vi "main.vi"() -> ()   [LabVIEW 2023]
uses:
  state-machine-states.ctl
  tab-control-states.ctl
  <vilib>/DAQmx/read.llb/DAQmx Read (Analog DBL 1Chan 1Samp).vi
  <vilib>/DAQmx/create/channels.llb/DAQmx Create Channel (AI-Temperature-Thermocouple).vi
  <vilib>/DAQmx/miscellaneous.llb/DAQmx Fill In Error Info.vi
  bronkhorst_flow-bus/Bronkhorst FLOW-BUS/Public/Data/Measure/Read Measure (Direct).vi
  bronkhorst_flow-bus/Bronkhorst FLOW-BUS/Public/Configure/Setpoint/Configure Setpoint (Percentage).vi
  bronkhorst_flow-bus/Bronkhorst FLOW-BUS/Public/Data/Setpoint/Read Setpoint (Percentage).vi
  bronkhorst_flow-bus/Bronkhorst FLOW-BUS/Public/Data/Measure/Read Measure (Percentage).vi
  bronkhorst_flow-bus/Bronkhorst FLOW-BUS/Bronkhorst FLOW-BUS.lvlib
panel:
  in  "Stop":bool
  in  "pause":bool
  in  "exit":bool
  out "state":T1
  out "error out":errorcluster
  out "Status":string
  in  "Tab Control":enum32{"setup", "run", "graphs", "errors"}(tab)
  in  "Start":bool
  in  "MFC 1":refnum<visa-resource-name>="COM31"
  in  "MFC 2":refnum<visa-resource-name>="COM32"
  in  "MFM 3":refnum<visa-resource-name>="COM33"
  in  "MFM 4":refnum<visa-resource-name>="COM34"
  in  "TC1 Channel":tag="cDAQ1Mod1/ai0"
  out "MFM4 (ml/min) 2":dbl caption="Measure Percentage"
  out "Measure (ml/min)":dbl caption="Measure Percentage"
  out "Measure (%) 2":dbl caption="Measure Percentage"
  in  "Setpoint  (%) 2":dbl min=0.0 max=100.0 step=1.0 format="%#.2g"
  out "Setpoint Percentage 2":dbl caption="Setpoint Percentage" format="%#g"
  out "Measure (%)":dbl caption="Measure Percentage"
  in  "Setpoint  (%)":dbl min=0.0 max=100.0 step=1.0 format="%#.2g"
  out "Setpoint Percentage":dbl format="%#g"
  out "TC1 (degC)":dbl format="%0.2f"
  out "MFM Sensor History":dbl[][](graph)
  out "Temperature Sensor History":dbl[](graph)
  out "errors":errorcluster
  in  "Clear Errors":bool
  # "Usage Instructions:\n\n1. Select \"setup\" tab, ensure correct \n    COM port & Channel for each device\n\n2. To start Data Aquisition press \"Start\" button\n\n3. Select Setpoint for MFC1 & MFC2\n\n4. View Graphs in \"graphs\" tab\n\n5. Pause and Unpause data aquisition with \"pause\" button\n\n6. To export data to Excel, right click on topmost graph view \n     and select:\n     - \"Export\" -> \"Export  Data to Excel\"\n     - Name & Save Excel file\n        (Note: All data will be exported not just \"active\" plots)\n\n\n7. To Clear sensor history press \"Stop\" button\n     - While stopped, setup controls are available\n\n8. To Exit program, click \"Exit\" Button\n\n9. If Error shows, attempt to remedy error then press\n     \"clear error\" button. Program will revert to Setup"
  # "Percentage"
  # "Gas  \nOut"
  # "Nitrogen \nIn"
  # "Ammonia \nIn"
  # "Gas  \nOut"
  # "MFC2"
  # "MFM4"
  # "MFM3"
  # "MFC1"
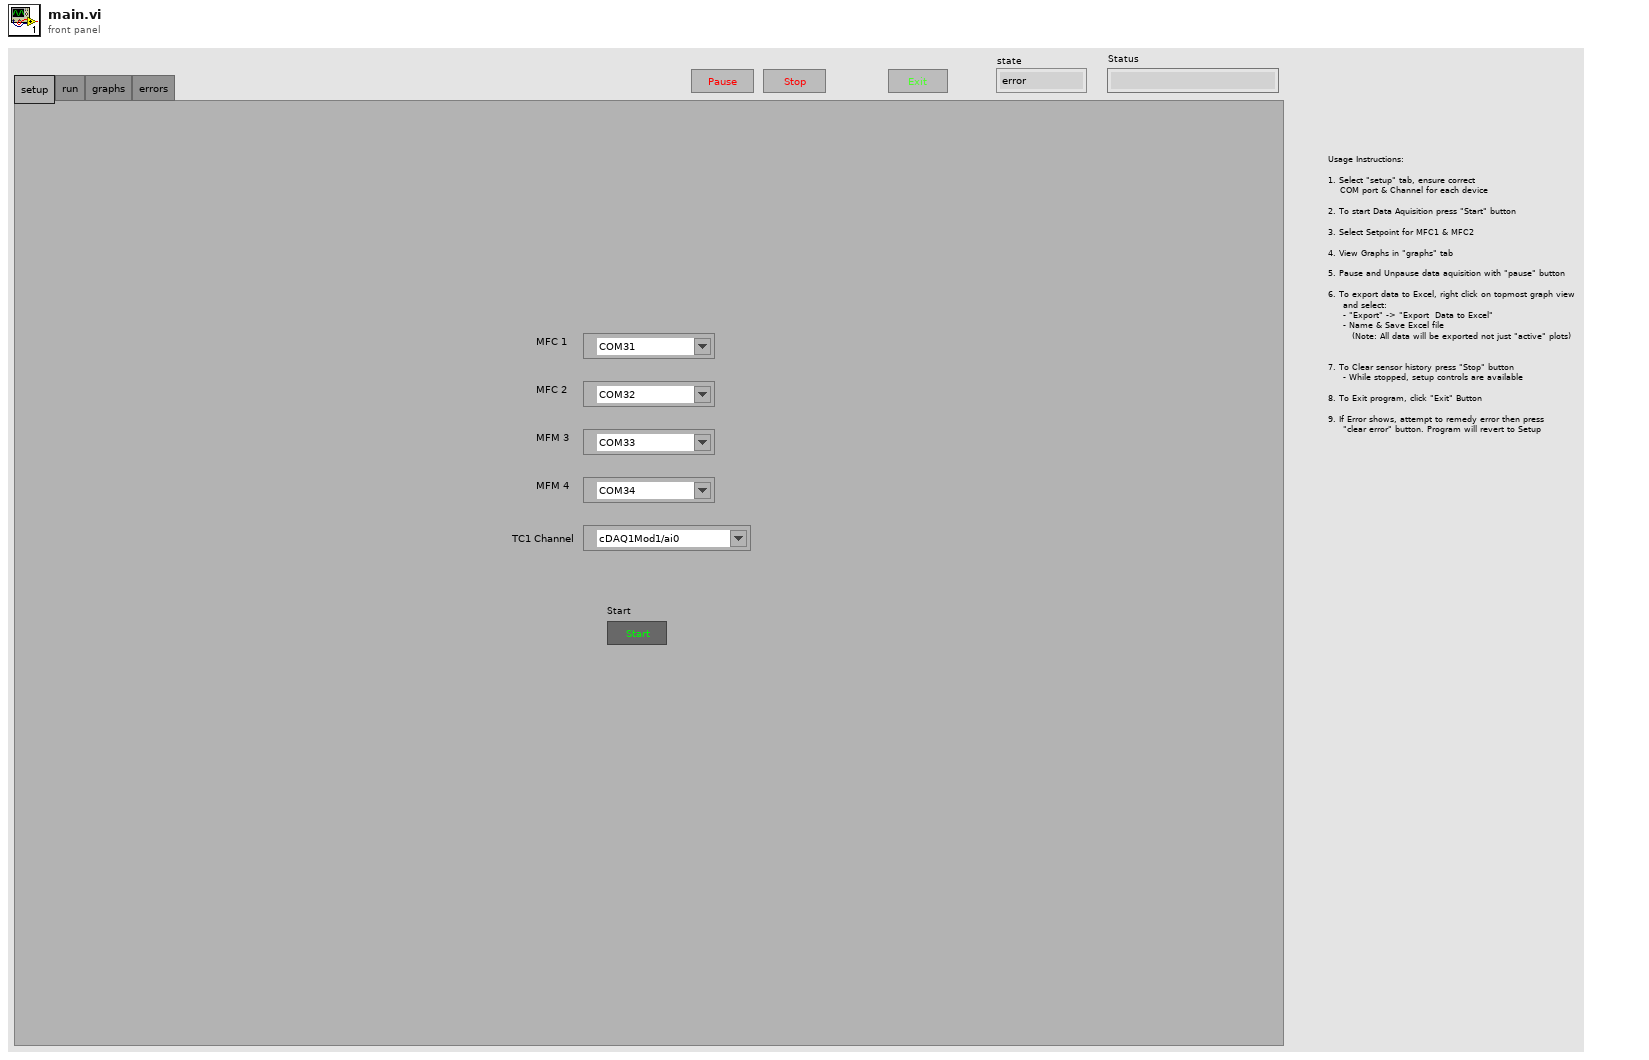
[diagram p1: front panel]
types:
  T1 = typedef "state-machine-states.ctl" = enum16{"error", "wait", "init", "start", "run", "stop", "clear-error", "shutdown"}
  T2 = enum8{"Enabled", "Disabled", "Disabled and Grayed Out"}
  T3 = typedef "tab-control-states.ctl" = enum32{"setup", "run", "graphs", "errors"}
  T4 = enum32{"BUS/RS232", "Analog input", "FLOW-BUS slave", "Valve close", "Controller idle", "Testing mode", "Tuning mode", "Setpoint 100%", "Valve fully open", "Calibration mode", "Analog slave", "Keyboard or FLOW-BUS setpoint", "Setpoint 0%", "FLOW-BUS analog slave", "(FPP) Range select mode", "(FPP) Manual start sensor select, automatic end sensor", "(FPP) Automatic start sensor select, manual end sensor", "(FPP) Automatic start and end sensor", "RS232 Setpoint", "RS232 broadcast mode", "Valve stearing (valve = setpoint)", "Analog valve stearing (valve = analog setpoint)", "Valve safe state"}
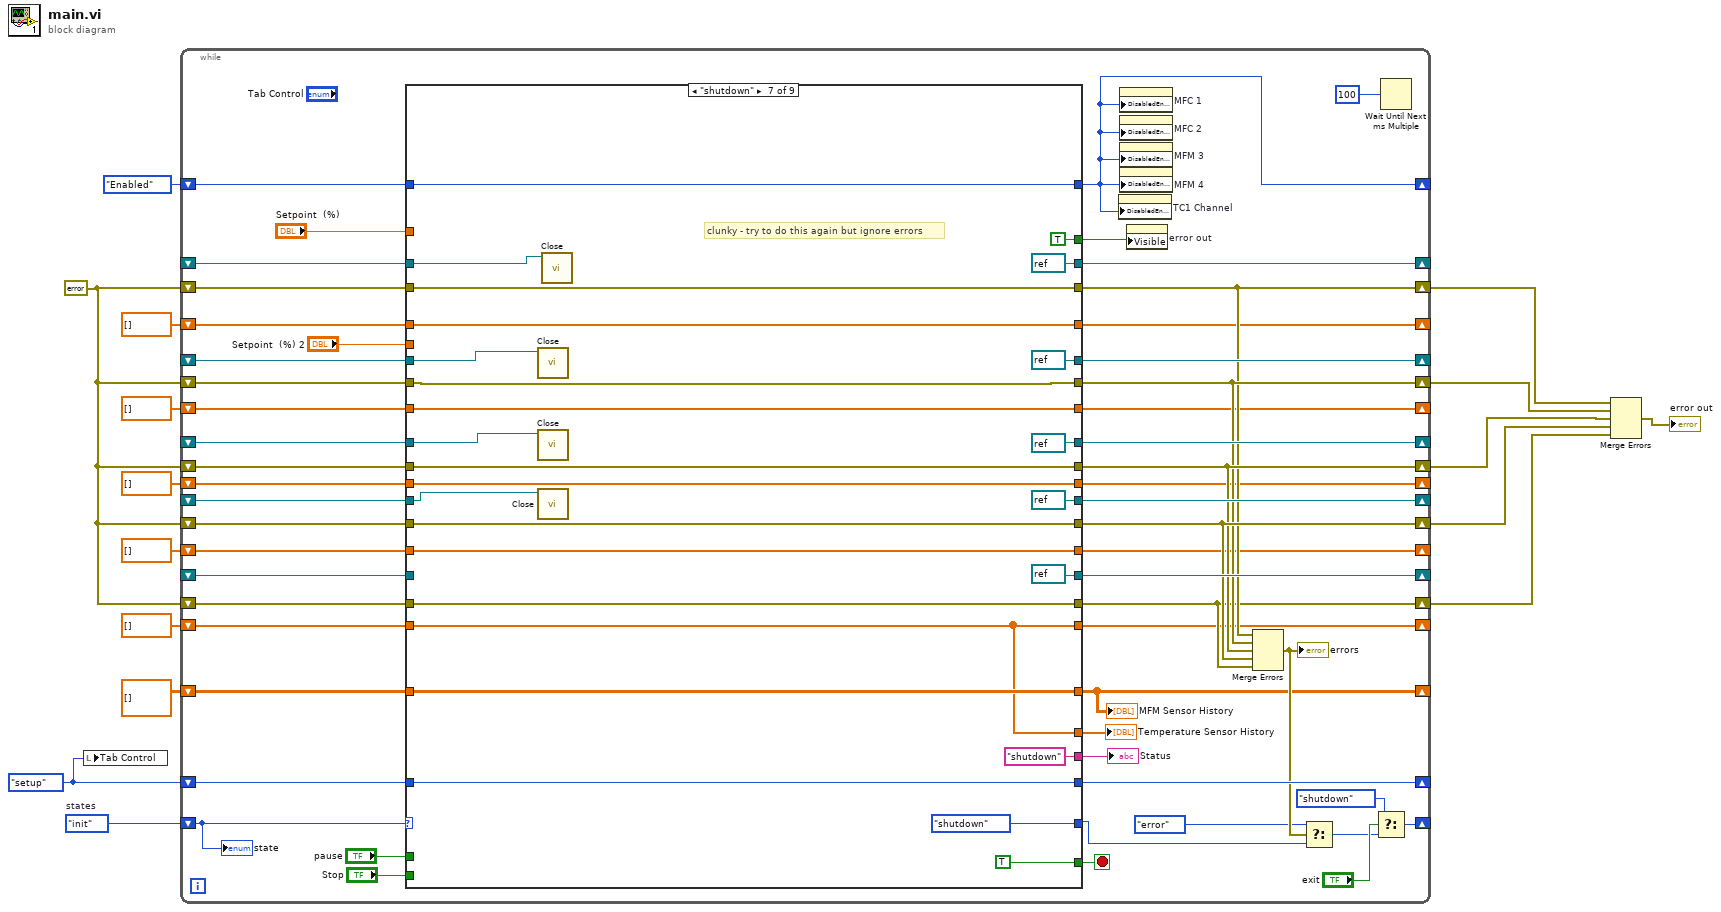
[diagram p0: block diagram]
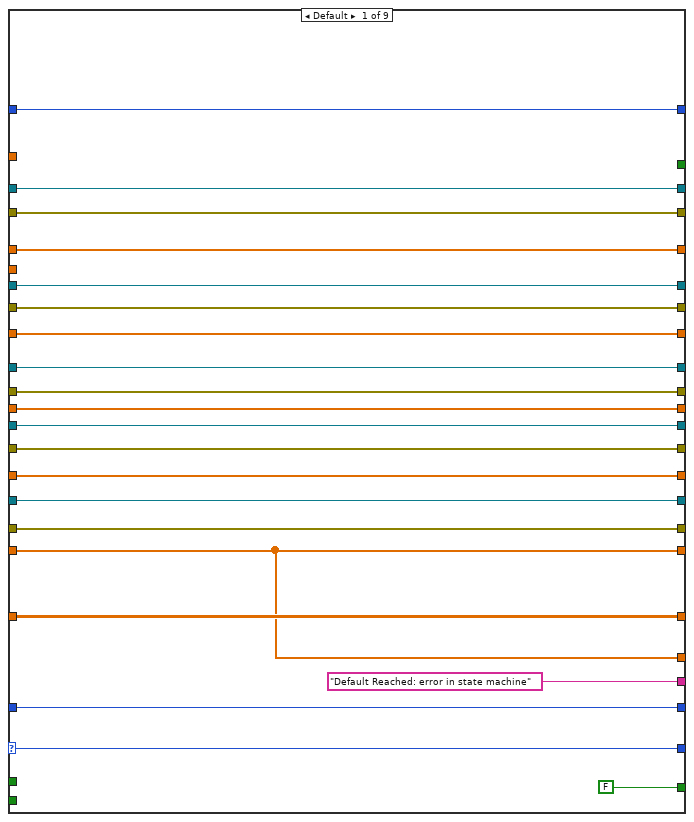
[diagram p2: hidden frame]
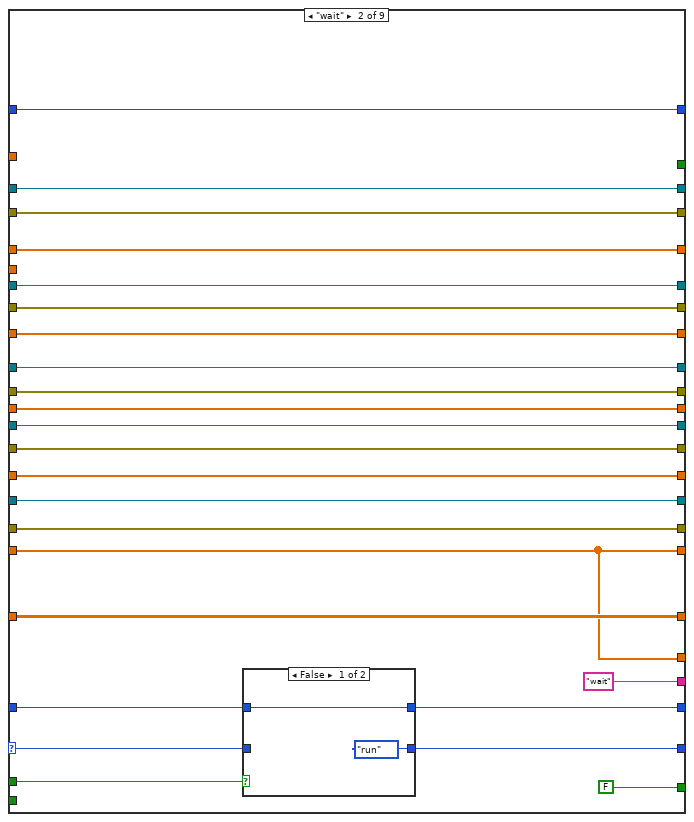
[diagram p3: hidden frame]
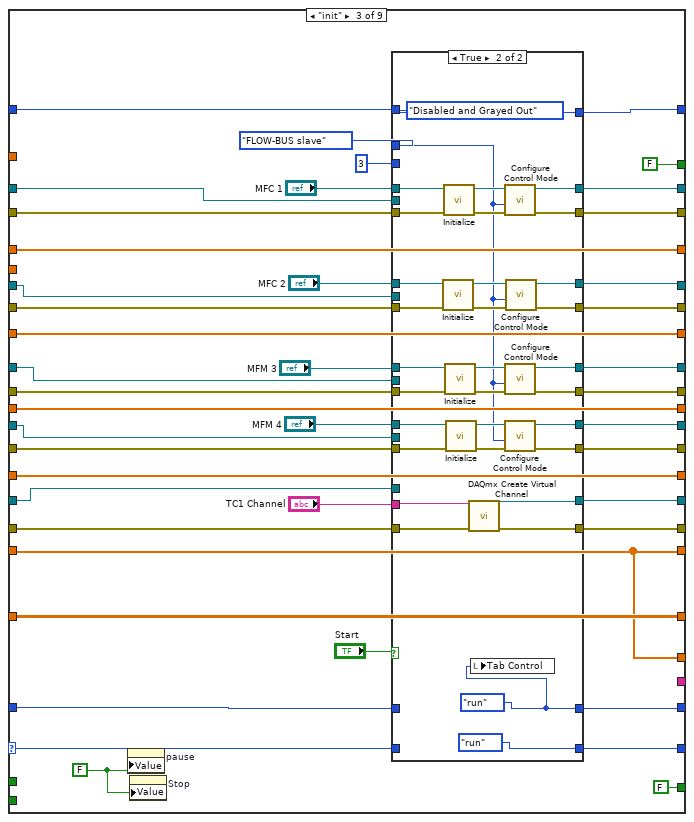
[diagram p5: hidden frame]
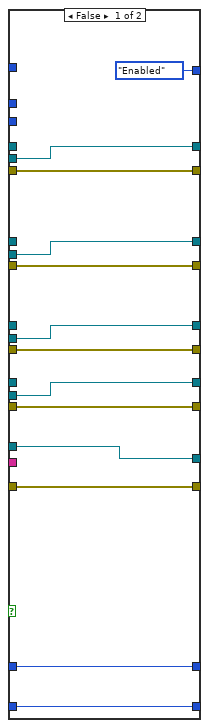
[diagram p6: hidden frame]
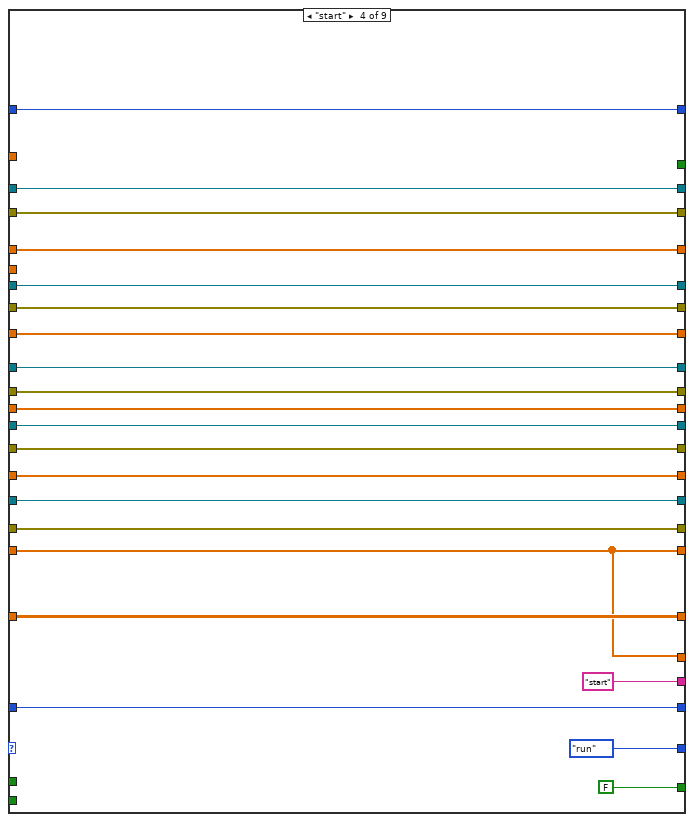
[diagram p7: hidden frame]
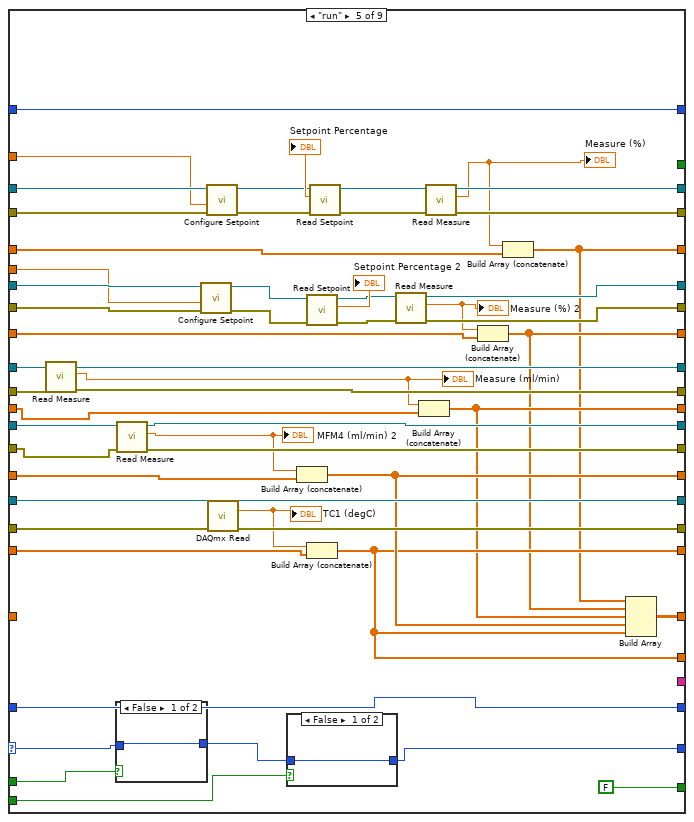
[diagram p8: hidden frame]
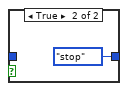
[diagram p9: hidden frame]
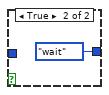
[diagram p10: hidden frame]
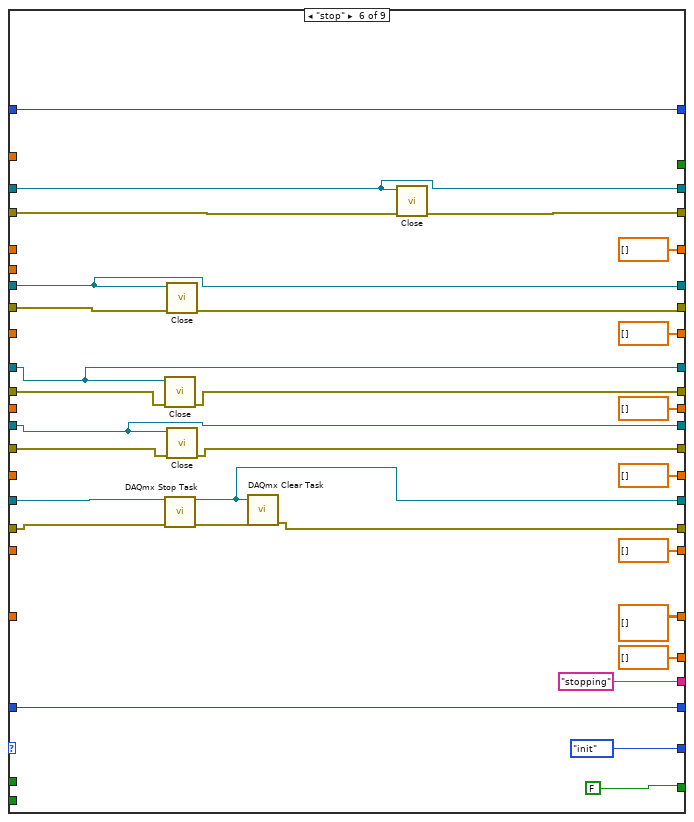
[diagram p11: hidden frame]
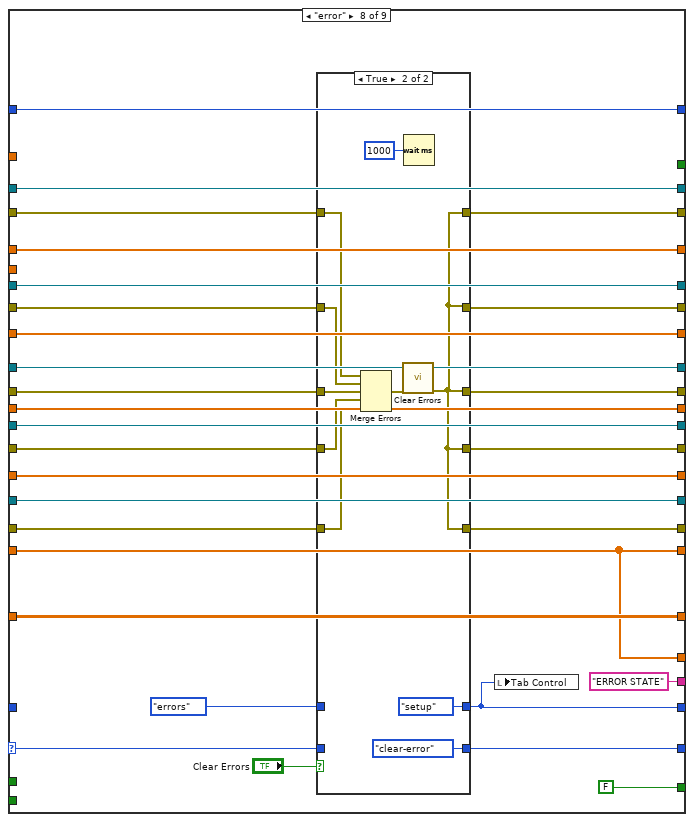
[diagram p12: hidden frame]
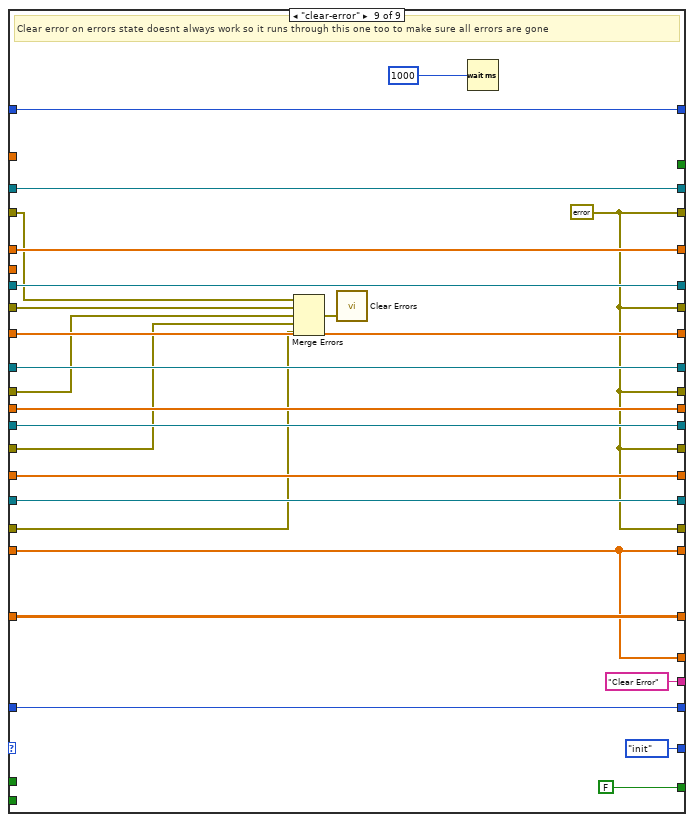
[diagram p14: hidden frame]
diagram:
  w9 = errorcluster {"status"=FALSE, "code"=0, "source"=""} ("error out")
  w10 = state-machine-states."init"  # states
  w7 = tab-control-states."setup" ("Tab Control")
  n1 = local write "Tab Control"(w7) -> ()
  n2 = while {
    shift-right: [w52] -> _
    shift-left: w7 -> [w39]
    shift-right: [w69] -> _
    shift-left: _ -> [w61]
    shift-right: [w44] -> w15
    shift-left: w9 -> [w65]
    shift-right: [w68] -> _
    shift-left: _ -> [w60]
    shift-right: [w45] -> w14
    shift-left: w9 -> [w64]
    shift-right: [w67] -> _
    shift-left: _ -> [w59]
    shift-right: [w46] -> w13
    shift-left: w9 -> [w63]
    shift-right: [w66] -> _
    shift-left: _ -> [w58]
    shift-right: [w47] -> w12
    shift-left: w9 -> [w62]
    shift-right: [w57] -> _
    shift-left: _ -> [w56]
    shift-right: [w43] -> w11
    shift-left: w9 -> [w55]
    shift-right: [w36] -> _
    shift-left: w10 -> [w50]
    shift-right: [w40] -> _
    shift-left: T2."Enabled" ("Disabled") -> [w41]
    shift-right: [w30] -> _
    shift-left: sgl[] [] -> [w29]
    shift-right: [w28] -> _
    shift-left: dbl[] [] -> [w27]
    shift-right: [w25] -> _
    shift-left: sgl[] [] -> [w24]
    shift-right: [w23] -> _
    shift-left: dbl[] [] -> [w22]
    shift-right: [w21] -> _
    shift-left: dbl[] [] -> [w20]
    shift-right: [w19] -> _
    shift-left: dbl[][] [] -> [w18]
    stop <- w34 stop-if-true
    n3 = case shown="\"shutdown\"" w50 {
      selector: w50 -> [w78 w98 w159 _ w251 _ _ w355 _]
      tunnel: [w80 w99 w127 w217 w248 w313 w341 w353 w389] -> w52
      tunnel: w39 -> [w80 w100 w160 w217 w248 w313 w341 _ w389]
      tunnel: [w90 w114 w139 w227 w272 w298 refnum<visa-resource-name> refnum ("VISA resource name out") w371 w412] -> w69
      tunnel: [w89 w113 w140 w226 w271 w315 w334 w347 w391] -> w44
      tunnel: [w87 w104 w145 w225 w266 w300 refnum<visa-resource-name> refnum ("VISA resource name out") w370 w411] -> w68
      tunnel: [w88 w105 w146 w224 w267 w301 w328 w346 w391] -> w45
      tunnel: [w86 w106 w151 w223 w258 w306 refnum<visa-resource-name> refnum ("VISA resource name out") w369 w410] -> w67
      tunnel: [w85 w107 w152 w222 w259 w307 w327 w345 w391] -> w46
      tunnel: [w84 w108 w155 w221 w255 w303 refnum<visa-resource-name> refnum ("VISA resource name out") w368 w409] -> w66
      tunnel: [w83 w109 w156 w220 w254 w302 w326 w344 w391] -> w47
      tunnel: w65 -> [w89 w113 w142 w226 w270 w299 w334 w352 w396]
      tunnel: w64 -> [w88 w105 w148 w224 w268 w305 w328 w351 w395]
      tunnel: w63 -> [w85 w107 w150 w222 w260 w308 w327 w350 w394]
      tunnel: w62 -> [w83 w109 w154 w220 w256 w304 w326 w349 w393]
      tunnel: w61 -> [w90 w114 w131 w227 w273 w298 w338 w371 w412]
      tunnel: w60 -> [w87 w104 w132 w225 w269 w300 w337 w370 w411]
      tunnel: w59 -> [w86 w106 w130 w223 w261 w306 w336 w369 w410]
      tunnel: w58 -> [w84 w108 w133 w221 w257 w303 w335 w368 w409]
      tunnel: [w82 w110 w135 w219 w263 w309 refnum<k21> refnum ("task out") w367 w408] -> w57
      tunnel: w56 -> [w82 w110 w138 w219 w265 w312 _ w367 w408]
      tunnel: [w81 w111 w134 w218 w262 w310 w325 w343 w391] -> w43
      tunnel: w55 -> [w81 w111 w136 w218 w264 w311 w325 w348 w392]
      tunnel: "Setpoint  (%)" -> [_ _ _ _ w253 _ _ _ _]
      tunnel: "Setpoint  (%) 2" -> [_ _ _ _ w252 _ _ _ _]
      tunnel: ["Default Reached: error in state machine" ("Status") "wait" ("Status") _ "start" ("Status") _ "stopping" ("Status") "shutdown" ("Status") "ERROR STATE" ("Status") "Clear Error" ("Status")] -> w51
      tunnel: [w78 w97 w158 state-machine-states."run" ("Enum") w244 state-machine-states."init" ("Enum") state-machine-states."shutdown" ("Enum") w356 state-machine-states."init"] -> w32
      tunnel: [FALSE ("x") FALSE ("x") FALSE ("x") FALSE ("x") FALSE ("x") FALSE ("x") TRUE ("x") FALSE ("x") FALSE ("x")] -> w34
      tunnel: [w76 w102 w129 w213 w249 w295 w339 w365 w406] -> w40
      tunnel: w41 -> [w76 w102 w128 w213 w249 w295 w339 w365 w406]
      tunnel: "pause" -> [_ w101 _ _ w247 _ _ _ _]
      tunnel: "Stop" -> [_ _ _ _ w246 _ _ _ _]
      tunnel: [w71 w92 w121 w212 w241 dbl[][] [] w323 w360 w401] -> w19
      tunnel: [w75 w94 w125 w211 w238 sgl[] [] w321 w361 w402] -> w30
      tunnel: w29 -> [w75 w94 w125 w211 w240 _ w321 w361 w402]
      tunnel: [w70 w91 w120 w207 w237 dbl[] [] w322 w359 w400] -> w28
      tunnel: w27 -> [w70 w91 w120 w207 w239 _ w322 w359 w400]
      tunnel: [w70 w91 w120 w207 w237 dbl[] [] w322 w359 w400] -> w26
      tunnel: [w74 w93 w124 w210 w230 sgl[] [] w320 w362 w403] -> w25
      tunnel: w24 -> [w74 w93 w124 w210 w235 _ w320 w362 w403]
      tunnel: [w73 w95 w123 w209 w229 dbl[] [] w319 w363 w404] -> w23
      tunnel: w22 -> [w73 w95 w123 w209 w233 _ w319 w363 w404]
      tunnel: [w72 w96 w122 w208 w228 dbl[] [] w318 w364 w405] -> w21
      tunnel: w20 -> [w72 w96 w122 w208 w232 _ w318 w364 w405]
      tunnel: w18 -> [w71 w92 w121 w212 _ _ w323 w360 w401]
      tunnel: [_ _ FALSE ("Visible") _ _ _ TRUE ("Visible") _ _] -> w17
      frame Default {
      }
      frame "wait" {
        n4 = case shown="False" w101 {
          tunnel: w98 -> [_ w117]
          tunnel: w100 -> [w116 w118]
          tunnel: [w116 w118] -> w99
          tunnel: [state-machine-states."run" w117] -> w97
          frame False {
          }
          frame True {
          }
        }
      }
      frame "init" {
        w126 = FALSE ("pause")
        n5 = property on="pause" class="Bool (strict)"("Value"=w126) -> ()  [unwired: 2 in, 2 out]
        n6 = property on="Stop" class="Bool (strict)"("Value"=w126) -> ()  [unwired: 2 in, 2 out]
        n7 = case shown="True" "Start" {
          tunnel: [w165 w175] -> w127
          tunnel: w160 -> [w165 _]
          tunnel: w159 -> [w164 _]
          tunnel: [w164 state-machine-states."run" ("Enum")] -> w158
          tunnel: [w169 w206] -> w156
          tunnel: [w174 w205] -> w155
          tunnel: w154 -> [w169 w204]
          tunnel: "MFM 4" -> [_ w203]
          tunnel: [w168 w200] -> w152
          tunnel: [w171 w199] -> w151
          tunnel: w150 -> [w168 w198]
          tunnel: "MFM 3" -> [_ w197]
          tunnel: w148 -> [w167 w192]
          tunnel: "MFC 2" -> [_ w191]
          tunnel: [w167 w190] -> w146
          tunnel: [w173 w189] -> w145
          tunnel: T4."FLOW-BUS slave" ("Control Mode (0: BUS/RS232)") -> [_ w179]
          tunnel: u8 3 ("Node (3)") -> [_ _]
          tunnel: w142 -> [w166 w186]
          tunnel: "MFC 1" -> [_ w185]
          tunnel: [w166 w184] -> w140
          tunnel: [w172 w183] -> w139
          tunnel: w138 -> [w162 _]
          tunnel: "TC1 Channel" -> [_ w177]
          tunnel: w136 -> [w170 w182]
          tunnel: [w162 w181] -> w135
          tunnel: [w170 w180] -> w134
          tunnel: w133 -> [w174 _]
          tunnel: w132 -> [w173 _]
          tunnel: w131 -> [w172 _]
          tunnel: w130 -> [w171 _]
          tunnel: [T2."Enabled" ("Disabled") T2."Disabled and Grayed Out" ("Disabled")] -> w129
          tunnel: w128 -> [_ _]
          frame False {
          }
          frame True {
            w175 = tab-control-states."run" ("Tab Control")
            n8 = call "Initialize.vi"("error in (no error)"=w192, "VISA resource name"=w191) -> ("error out"=w193:errorcluster, "VISA resource name out"=w194:refnum<visa-resource-name>)  [unwired: 8 in]
            n9 = call "Initialize.vi"("error in (no error)"=w186, "VISA resource name"=w185) -> ("error out"=w187:errorcluster, "VISA resource name out"=w188:refnum<visa-resource-name>)  [unwired: 8 in]
            n10 = call "Initialize.vi"("error in (no error)"=w198, "VISA resource name"=w197) -> ("error out"=w196:errorcluster, "VISA resource name out"=w195:refnum<visa-resource-name>)  [unwired: 8 in]
            n11 = call "Initialize.vi"("error in (no error)"=w204, "VISA resource name"=w203) -> ("error out"=w202:errorcluster, "VISA resource name out"=w201:refnum<visa-resource-name>)  [unwired: 8 in]
            n12 = call-poly <vilib>:"DAQmx Create Virtual Channel.vi"("physical channels"=w177, "error in"=w182) -> ("task out"=w181:refnum<k21>, "error out"=w180:errorcluster)  [unwired: 12 in]
            n13 = local write "Tab Control"(w175) -> ()
            n14 = call "Configure Control Mode.vi"("error in (no error)"=w187, "Control Mode (0: BUS/RS232)"=w179, "VISA resource name"=w188) -> ("error out"=w184:errorcluster, "VISA resource name out"=w183:refnum<visa-resource-name>)  [unwired: 7 in]
            n15 = call "Configure Control Mode.vi"("error in (no error)"=w196, "Control Mode (0: BUS/RS232)"=w179, "VISA resource name"=w195) -> ("error out"=w200:errorcluster, "VISA resource name out"=w199:refnum<visa-resource-name>)  [unwired: 7 in]
            n16 = call "Configure Control Mode.vi"("error in (no error)"=w202, "Control Mode (0: BUS/RS232)"=w179, "VISA resource name"=w201) -> ("error out"=w206:errorcluster, "VISA resource name out"=w205:refnum<visa-resource-name>)  [unwired: 7 in]
            n17 = call "Configure Control Mode.vi"("error in (no error)"=w193, "Control Mode (0: BUS/RS232)"=w179, "VISA resource name"=w194) -> ("error out"=w190:errorcluster, "VISA resource name out"=w189:refnum<visa-resource-name>)  [unwired: 7 in]
          }
        }
      }
      frame "start" {
      }
      frame "run" {
        n18 = call-poly "Read Measure.vi"("error in (no error)"=w260, "VISA resource name"=w261) -> ("error out"=w259:errorcluster, "Measure Direct"=w236:sgl, "VISA resource name out"=w258:refnum<visa-resource-name>)  [unwired: 7 in]
        "Measure (ml/min)" <- w236
        n19 = case shown="False" w247 {
          tunnel: w251 -> [w286 _]
          tunnel: [w286 state-machine-states."wait"] -> w245
          frame False {
          }
          frame True {
          }
        }
        n20 = call-poly "Read Measure.vi"("error in (no error)"=w256, "VISA resource name"=w257) -> ("error out"=w254:errorcluster, "Measure Direct"=w243:sgl, "VISA resource name out"=w255:refnum<visa-resource-name>)  [unwired: 7 in]
        "MFM4 (ml/min) 2" <- w243
        n21 = call-poly "Configure Setpoint.vi"("error in (no error)"=w268, "Setpoint Percentage (0%)"=w252, "VISA resource name"=w269) -> ("error out"=w280:errorcluster, "VISA resource name out"=w279:refnum<visa-resource-name>)  [unwired: 7 in]
        n22 = call-poly "Configure Setpoint.vi"("error in (no error)"=w270, "Setpoint Percentage (0%)"=w253, "VISA resource name"=w273) -> ("error out"=w276:errorcluster, "VISA resource name out"=w274:refnum<visa-resource-name>)  [unwired: 7 in]
        n23 = call-poly <vilib>:"DAQmx Read.vi"("task/channels in"=w265, "error in"=w264) -> ("task out"=w263:refnum<k21>, "data"=w242:dbl, "error out"=w262:errorcluster)  [unwired: 11 in]
        "TC1 (degC)" <- w242
        n24 = case shown="False" w246 {
          tunnel: w245 -> [w284 _]
          tunnel: [w284 state-machine-states."stop"] -> w244
          frame False {
          }
          frame True {
          }
        }
        n25 = Build Array (concatenate)(w243, w240) -> (w238:sgl[])
        n26 = call-poly "Read Setpoint.vi"("error in (no error)"=w280, "VISA resource name"=w279) -> ("error out"=w282:errorcluster, "Setpoint Percentage"=→"Setpoint Percentage 2":dbl, "VISA resource name out"=w281:refnum<visa-resource-name>)  [unwired: 7 in]
        n27 = Build Array (concatenate)(w242, w239) -> (w237:dbl[])
        n28 = call-poly "Read Setpoint.vi"("error in (no error)"=w276, "VISA resource name"=w274) -> ("error out"=w278:errorcluster, "Setpoint Percentage"=→"Setpoint Percentage":dbl, "VISA resource name out"=w277:refnum<visa-resource-name>)  [unwired: 7 in]
        n29 = call-poly "Read Measure.vi"("error in (no error)"=w282, "VISA resource name"=w281) -> ("error out"=w267:errorcluster, "Measure Percentage"=w234:dbl, "VISA resource name out"=w266:refnum<visa-resource-name>)  [unwired: 7 in]
        "Measure (%) 2" <- w234
        n30 = Build Array (concatenate)(w236, w235) -> (w230:sgl[])
        n31 = call-poly "Read Measure.vi"("error in (no error)"=w278, "VISA resource name"=w277) -> ("error out"=w271:errorcluster, "Measure Percentage"=w231:dbl, "VISA resource name out"=w272:refnum<visa-resource-name>)  [unwired: 7 in]
        "Measure (%)" <- w231
        n32 = Build Array (concatenate)(w234, w233) -> (w229:dbl[])
        n33 = Build Array (concatenate)(w231, w232) -> (w228:dbl[])
        n34 = Build Array(w228, w229, w230, w238, w237) -> (w241:dbl[][])
      }
      frame "stop" {
        n35 = call "Close.vi"("error in (no error)"=w308, "VISA resource name"=w306) -> ("error out"=w307:errorcluster)  [unwired: 9 in]
        n36 = call <vilib>:"DAQmx Stop Task.vi"("task/channels in"=w312, "error in"=w311) -> ("task out"=w309:refnum<k21>, "error out"=w316:errorcluster)  [unwired: 12 in]
        n37 = call "Close.vi"("error in (no error)"=w305, "VISA resource name"=w300) -> ("error out"=w301:errorcluster)  [unwired: 9 in]
        n38 = call "Close.vi"("error in (no error)"=w304, "VISA resource name"=w303) -> ("error out"=w302:errorcluster)  [unwired: 9 in]
        n39 = call <vilib>:"DAQmx Clear Task.vi"("task in"=w309, "error in"=w316) -> ("error out"=w310:errorcluster)  [unwired: 13 in]
        n40 = call "Close.vi"("error in (no error)"=w299, "VISA resource name"=w298) -> ("error out"=w315:errorcluster)  [unwired: 9 in]
      }
      frame "shutdown" {
        # "clunky - try to do this again but ignore errors"
        n41 = call "Close.vi"("VISA resource name"=w337) -> ()  [unwired: 10 in, 1 out]
        n42 = call "Close.vi"("VISA resource name"=w336) -> ()  [unwired: 10 in, 1 out]
        n43 = call "Close.vi"("VISA resource name"=w335) -> ()  [unwired: 10 in, 1 out]
        n44 = call "Close.vi"("VISA resource name"=w338) -> ()  [unwired: 10 in, 1 out]
      }
      frame "error" {
        n45 = case shown="True" "Clear Errors" {
          tunnel: [w377 state-machine-states."clear-error"] -> w356
          tunnel: w355 -> [w377 _]
          tunnel: tab-control-states."errors" ("Tab Control") -> [w378 _]
          tunnel: [w378 tab-control-states."setup" ("Tab Control")] -> w353
          tunnel: w352 -> [w376 w386]
          tunnel: w351 -> [w375 w385]
          tunnel: w350 -> [w374 w384]
          tunnel: w349 -> [w373 w383]
          tunnel: w348 -> [w372 w382]
          tunnel: [w376 w380] -> w347
          tunnel: [w375 w380] -> w346
          tunnel: [w374 w380] -> w345
          tunnel: [w373 w380] -> w344
          tunnel: [w372 w380] -> w343
          frame False {
          }
          frame True {
            n46 = Merge Errors(w386, w385, w384, w383, w382) -> (w381:errorcluster)
            n47 = call <vilib>:"Clear Errors.vi"("error in (no error)"=w381) -> ("error out"=w380:errorcluster)  [unwired: 5 in, 1 out]
            n48 = Wait (ms)(milliseconds to wait=u32 1000) -> ()  [unwired: 1 out]
          }
        }
        n49 = local write "Tab Control"(w353) -> ()
      }
      frame "clear-error" {
        w391 = errorcluster {"status"=FALSE, "code"=0, "source"=""} ("error out")
        # "Clear error on errors state doesnt always work so it runs through this one too to make sure all errors are gone"
        n50 = Merge Errors(w396, w395, w394, w393, w392) -> (w398:errorcluster)
        n51 = call <vilib>:"Clear Errors.vi"("error in (no error)"=w398) -> ()  [unwired: 5 in, 2 out]
        n52 = Wait (ms)(milliseconds to wait=u32 1000) -> ()  [unwired: 1 out]
      }
    }
    "Status" <- w51
    "MFM Sensor History" <- w19
    "Temperature Sensor History" <- w26
    n53 = property on="TC1 Channel" class="DAQmxName"("DisabledEnum"=w40) -> ()  [unwired: 2 in, 2 out]
    n54 = property on="MFC 1" class="VISAName"("DisabledEnum"=w40) -> ()  [unwired: 2 in, 2 out]
    n55 = property on="MFC 2" class="VISAName"("DisabledEnum"=w40) -> ()  [unwired: 2 in, 2 out]
    n56 = property on="MFM 3" class="VISAName"("DisabledEnum"=w40) -> ()  [unwired: 2 in, 2 out]
    n57 = property on="MFM 4" class="VISAName"("DisabledEnum"=w40) -> ()  [unwired: 2 in, 2 out]
    n58 = property on="error out" class="Clust (strict)"("Visible"=w17) -> ()  [unwired: 2 in, 2 out]
    n59 = Merge Errors(w44, w45, w46, w47, w43) -> (w49:errorcluster)
    "errors" <- w49
    n60 = Select(t=state-machine-states."error", s=w49, f=w32) -> (s? t:f=w31:T1)
    n61 = Select(t=state-machine-states."shutdown", s="exit", f=w31) -> (s? t:f=w36:T1)
    n62 = Wait Until Next ms Multiple(millisecond multiple=u32 100) -> ()  [unwired: 1 out]
    "state" <- w50
  }
  n63 = Merge Errors(w15, w14, w13, w12, w11) -> (→"error out":errorcluster)
